vi "Interface.RT FIFO.Write.16B.vi"(6 "overwrite on timeout (T)":bool, 7 "FIFO Debug Flags":refnum<class "FIFO Flags.lvclass">, 8 "error in (no error)":errorcluster, 9 "timeout in ms (0)":i32, 10 "element":T2, 11 "RT FIFO in":T1) -> (0 "error out":errorcluster, 1 "timed out?":bool, 3 "RT FIFO out":T1)   [LabVIEW 2017, in "DSF Core.lvlib" / "Interface.lvclass"]
uses:
  Interface.lvclass
  Interface.RT FIFO.Data.16B.ctl
  Interface.RT FIFO.Payload.16B.ctl
  Interface.RT FIFO.Ref.16B.ctl
  Debug/FIFO Flags.lvclass
  Debug/FIFO Flags.lvclass/FIFO Flags.ctl
panel:
  out "# elements":u32
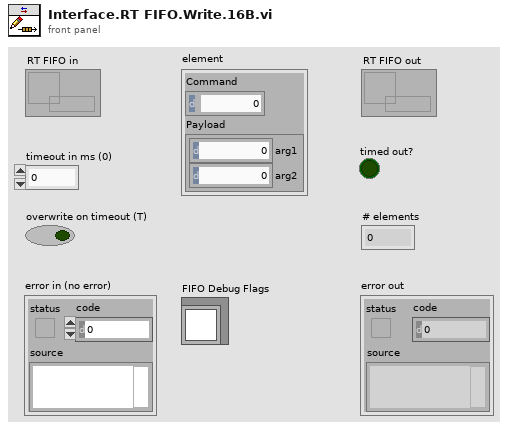
[diagram p1: front panel]
types:
  T1 = typedef "DSF Core.lvlib/Interface.lvclass/Interface.RT FIFO.Ref.16B.ctl" = refnum<k33>
  T2 = typedef "DSF Core.lvlib/Interface.lvclass/Interface.RT FIFO.Data.16B.ctl" = cluster{"Command":u8, "Payload":T3}
  T3 = typedef "DSF Core.lvlib/Interface.lvclass/Interface.RT FIFO.Payload.16B.ctl" = cluster{"arg1":u64, "arg2":u64}
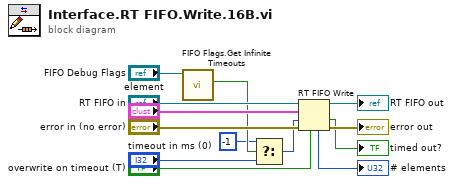
[diagram p0: block diagram]
diagram:
  n1 = call "FIFO Flags.Get Infinite Timeouts.vi"("FIFO Debug Flags in"="FIFO Debug Flags") -> ("infinite timeouts"=w5:bool)  [unwired: 9 in, 1 out]
  n2 = Select(t=-1, s=w5, f="timeout in ms (0)") -> (s? t:f=w3:i32)
  n3 = RT FIFO Write(0:"RT FIFO in", 1:"element", 2:w3, 3:"error in (no error)", 5:"overwrite on timeout (T)") -> (7:→"# elements":u32, 8:→"RT FIFO out":T1, 10:→"timed out?":bool, 11:→"error out":errorcluster)
